vi "Read Directory Path.vi"(8 "error in (no error)":errorcluster, 11 "MeasurementSMO in":refnum<class "AFM_Litho_Plugin.IV.lvclass">) -> (0 "error out":errorcluster, 2 "Directory Path":path, 3 "MeasurementSMO out":refnum<class "AFM_Litho_Plugin.IV.lvclass">)   [LabVIEW 2019, in "AFM_Litho_Plugin.IV.lvclass"]
uses:
  AFM_Litho_Plugin.IV.lvclass
  AFM_Litho_Plugin.IV.lvclass/AFM_Litho_Plugin.IV.ctl
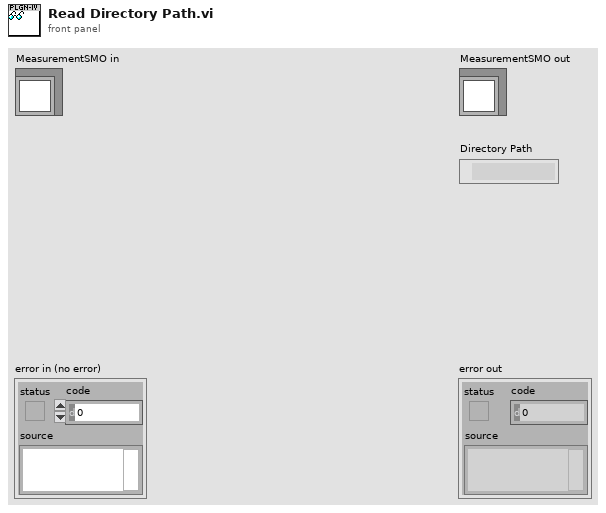
[diagram p1: front panel]
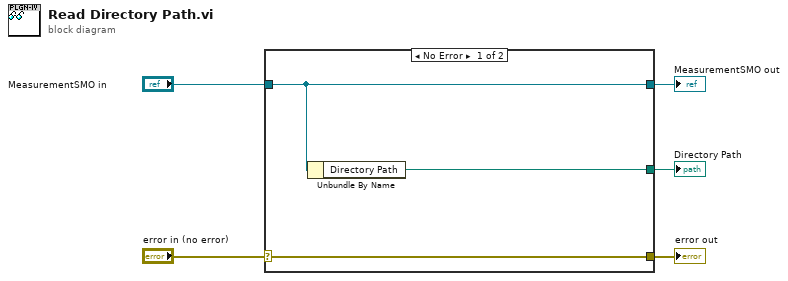
[diagram p0: block diagram]
diagram:
  n1 = case shown="No Error" "error in (no error)" {
    selector: "error in (no error)" -> [w8 w9]
    tunnel: [w8 w9] -> w4
    tunnel: [w7 w10] -> w2
    tunnel: "MeasurementSMO in" -> [w7 w10]
    tunnel: [w6 _] -> w1
    frame No Error {
      n2 = Unbundle By Name(w7) -> ("Directory Path"=w6:path)
    }
    frame Error {
    }
  }
  "error out" <- w4
  "MeasurementSMO out" <- w2
  "Directory Path" <- w1
